vi "BRig_Host__Loop_Producer__tcp_System__Data_v2.vi"(0 "input_strCmd":string) -> ()   [LabVIEW 2014]
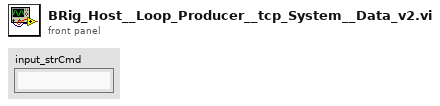
[diagram p1: front panel]
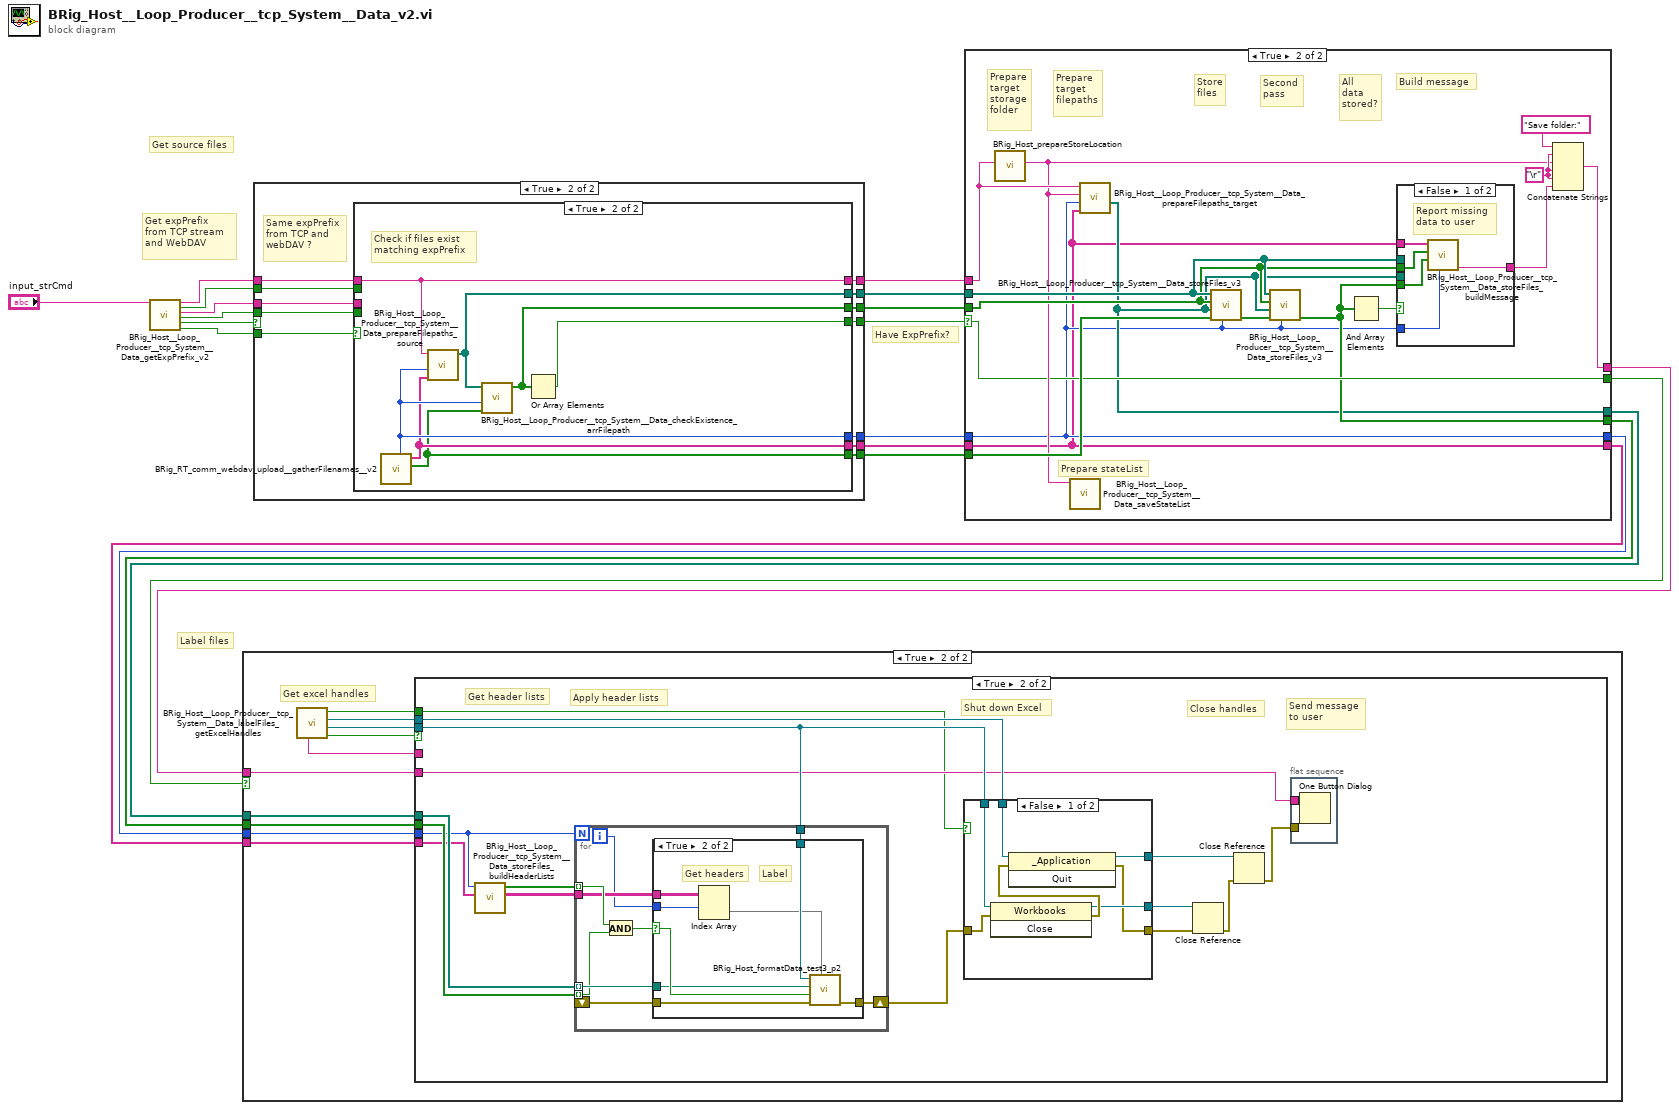
[diagram p0: block diagram]
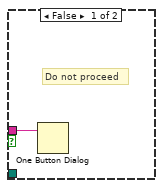
[diagram p2: hidden frame]
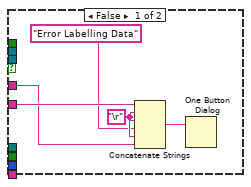
[diagram p3: hidden frame]
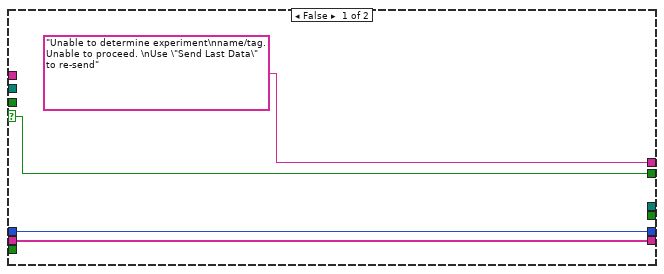
[diagram p6: hidden frame]
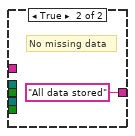
[diagram p7: hidden frame]
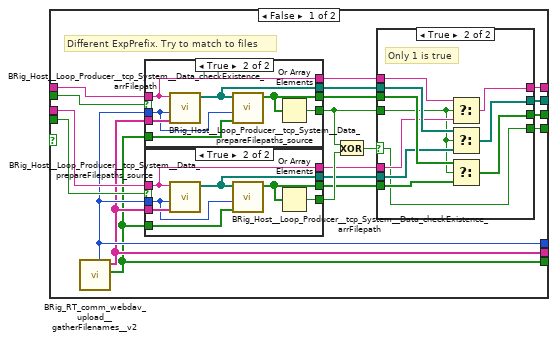
[diagram p9: hidden frame]
diagram:
  # "Label files"
  # "Have ExpPrefix?"
  # "Get expPrefix\nfrom TCP stream\nand WebDAV"
  # "Get source files"
  n1 = call "BRig_Host__Loop_Producer__tcp_System__Data_getExpPrefix_v2.vi"("input_strCmd"="input_strCmd") -> (14:"output_expPrefix_tcp"=w14:string, 15:"output_expPrefix_tcp"=w15:bool, 16:"output_expPrefix_webdav"=w16:string, 17:"output_expPrefix_webdav"=w17:bool, "output_expPrefix_any"=w19:bool, "output_expPrefix_same"=w18:bool)  [unwired: 13 in]
  n2 = case shown="True" w19 {
    tunnel: w18 -> [_ w32]
    tunnel: w17 -> [_ w28]
    tunnel: w16 -> [_ w30]
    tunnel: w15 -> [_ w29]
    tunnel: w14 -> [_ w31]
    tunnel: [_ w27] -> w12
    tunnel: [_ w26] -> w11
    tunnel: [_ w25] -> w10
    tunnel: [_ w24] -> w13
    tunnel: [_ w23] -> w9
    tunnel: [_ w22] -> w8
    tunnel: [_ w21] -> w7
    frame False {
    }
    frame True {
      # "Same expPrefix\nfrom TCP and\nwebDAV ?"
      n3 = case shown="True" w32 {
        tunnel: w31 -> [w51 w84]
        tunnel: w30 -> [w50 _]
        tunnel: w29 -> [w52 _]
        tunnel: w28 -> [w49 _]
        tunnel: [w39 w84] -> w27
        tunnel: [w38 w83] -> w26
        tunnel: [w37 w82] -> w25
        tunnel: [w36 w81] -> w24
        tunnel: [w35 w80] -> w23
        tunnel: [w34 w79] -> w22
        tunnel: [w33 w78] -> w21
        frame False {
          # "Different ExpPrefix. Try to match to files"
          n4 = call "BRig_RT_comm_webdav_upload__gatherFilenames__v2.vi"() -> ("output_arrBlank"=w33:bool[], "output_arrFilenames"=w34:string[], "output_n"=w35:i32)  [unwired: 9 in]
          n5 = case shown="True" w52 {
            tunnel: w51 -> [_ w74]
            tunnel: w35 -> [_ w76]
            tunnel: w34 -> [_ w77]
            tunnel: w33 -> [_ w75]
            tunnel: [_ w74] -> w46
            tunnel: [_ w73] -> w45
            tunnel: [_ w72] -> w44
            tunnel: [_ w71] -> w40
            frame False {
            }
            frame True {
              n6 = call "BRig_Host__Loop_Producer__tcp_System__Data_prepareFilepaths_source.vi"("input_arrFilenames"=w77, "input_nFilenames"=w76, "input_expPrefix"=w74) -> ("output_arrPath"=w73:path[])  [unwired: 8 in]
              n7 = call "BRig_Host__Loop_Producer__tcp_System__Data_checkExistence_arrFilepath.vi"("input_I_arrPath"=w75, "input_n"=w76, "input_arrPath"=w73) -> ("output_exist"=w72:bool[])  [unwired: 8 in]
              n8 = Or Array Elements(Boolean array=w72) -> (logical OR=w71:bool)
            }
          }
          n9 = case shown="True" w49 {
            tunnel: w50 -> [_ w67]
            tunnel: w35 -> [_ w69]
            tunnel: w34 -> [_ w70]
            tunnel: w33 -> [_ w68]
            tunnel: [_ w67] -> w43
            tunnel: [_ w66] -> w42
            tunnel: [_ w65] -> w41
            tunnel: [_ w64] -> w48
            frame False {
            }
            frame True {
              n10 = call "BRig_Host__Loop_Producer__tcp_System__Data_prepareFilepaths_source.vi"("input_arrFilenames"=w70, "input_nFilenames"=w69, "input_expPrefix"=w67) -> ("output_arrPath"=w66:path[])  [unwired: 8 in]
              n11 = call "BRig_Host__Loop_Producer__tcp_System__Data_checkExistence_arrFilepath.vi"("input_I_arrPath"=w68, "input_n"=w69, "input_arrPath"=w66) -> ("output_exist"=w65:bool[])  [unwired: 8 in]
              n12 = Or Array Elements(Boolean array=w65) -> (logical OR=w64:bool)
            }
          }
          n13 = Exclusive Or(1:w48, 2:w40) -> (0:w47:bool)
          n14 = case shown="True" w47 {
            selector: w47 -> [_ w53]
            tunnel: w46 -> [_ w63]
            tunnel: w45 -> [_ w62]
            tunnel: w44 -> [_ w61]
            tunnel: w43 -> [_ w60]
            tunnel: w42 -> [_ w59]
            tunnel: w41 -> [_ w58]
            tunnel: w40 -> [_ w57]
            tunnel: [_ w56] -> w39
            tunnel: [_ w55] -> w38
            tunnel: [_ w54] -> w37
            tunnel: [_ w53] -> w36
            frame False {
              # "Both false or both true\n\nIf false, can't proceed\nIf true, no way to choose"
            }
            frame True {
              # "Only 1 is true"
              n15 = Select(t=w63, s=w57, f=w60) -> (s? t:f=w56:string)
              n16 = Select(t=w62, s=w57, f=w59) -> (s? t:f=w55:path[])
              n17 = Select(t=w61, s=w57, f=w58) -> (s? t:f=w54:bool[])
            }
          }
        }
        frame True {
          # "Check if files exist\nmatching expPrefix"
          n18 = call "BRig_RT_comm_webdav_upload__gatherFilenames__v2.vi"() -> ("output_arrBlank"=w78:bool[], "output_arrFilenames"=w79:string[], "output_n"=w80:i32)  [unwired: 9 in]
          n19 = call "BRig_Host__Loop_Producer__tcp_System__Data_prepareFilepaths_source.vi"("input_arrFilenames"=w79, "input_nFilenames"=w80, "input_expPrefix"=w84) -> ("output_arrPath"=w83:path[])  [unwired: 8 in]
          n20 = call "BRig_Host__Loop_Producer__tcp_System__Data_checkExistence_arrFilepath.vi"("input_I_arrPath"=w78, "input_n"=w80, "input_arrPath"=w83) -> ("output_exist"=w82:bool[])  [unwired: 8 in]
          n21 = Or Array Elements(Boolean array=w82) -> (logical OR=w81:bool)
        }
      }
    }
  }
  n22 = case shown="True" w13 {
    selector: w13 -> [w87 w93]
    tunnel: w12 -> [_ w104]
    tunnel: w11 -> [_ w100]
    tunnel: w10 -> [_ w99]
    tunnel: w9 -> [w85 w90]
    tunnel: w8 -> [w86 w89]
    tunnel: w7 -> [_ w103]
    tunnel: ["Unable to determine experiment\nname/tag. Unable to proceed. \nUse \"Send Last Data\" to re-send" ("message") w94] -> w3
    tunnel: [w87 w93] -> w4
    tunnel: [_ w92] -> w6
    tunnel: [_ w91] -> w5
    tunnel: [w85 w90] -> w2
    tunnel: [w86 w89] -> w1
    frame False {
    }
    frame True {
      w98 = "\r"
      # "Build message"
      # "All\ndata\nstored?"
      # "Second\npass"
      # "Store\nfiles"
      # "Prepare stateList"
      # "Prepare\ntarget\nstorage\nfolder"
      # "Prepare\ntarget\nfilepaths"
      n23 = call "BRig_Host_prepareStoreLocation.vi"("input_expPrefix"=w104) -> ("output_folderPath"=w97:string)  [unwired: 9 in, 1 out]
      n24 = call "BRig_Host__Loop_Producer__tcp_System__Data_saveStateList.vi"("input_filepath_storage"=w97) -> ()  [unwired: 11 in]
      n25 = call "BRig_Host__Loop_Producer__tcp_System__Data_prepareFilepaths_target.vi"("input_arrFilenames"=w89, "input_nFilenames"=w90, "input_storagePath"=w97, "input_expPrefix"=w104) -> ("output_arrPath_target"=w91:path[])  [unwired: 7 in]
      n26 = call "BRig_Host__Loop_Producer__tcp_System__Data_storeFiles_v3.vi"("input_n"=w90, "input_stored"=w103, "input_arrPath_target"=w91, "input_exist_source"=w99, "input_arrPath_source"=w100) -> ("output_stored"=w102:bool[])  [unwired: 6 in]
      n27 = call "BRig_Host__Loop_Producer__tcp_System__Data_storeFiles_v3.vi"("input_n"=w90, "input_stored"=w102, "input_arrPath_target"=w91, "input_exist_source"=w99, "input_arrPath_source"=w100) -> ("output_stored"=w92:bool[])  [unwired: 6 in]
      n28 = And Array Elements(Boolean array=w92) -> (logical AND=w101:bool)
      n29 = case shown="False" w101 {
        tunnel: w100 -> [_ _]
        tunnel: w99 -> [w108 _]
        tunnel: w91 -> [_ _]
        tunnel: w92 -> [w107 _]
        tunnel: w89 -> [w109 _]
        tunnel: w90 -> [w106 _]
        tunnel: [w105 "All data stored" ("output_msg")] -> w95
        frame False {
          # "Report missing\ndata to user"
          n30 = call "BRig_Host__Loop_Producer__tcp_System__Data_storeFiles_buildMessage.vi"("input_n"=w106, "input_stored"=w107, "input_exist_source"=w108, "input_arrFilenames"=w109) -> ("output_msg"=w105:string)  [unwired: 7 in]
        }
        frame True {
          # "No missing data"
        }
      }
      n31 = Concatenate Strings("Save folder:" ("string"), w98, w97, w98, w98, w95) -> (w94:string)
    }
  }
  n32 = case shown="True" w4 {
    tunnel: w6 -> [_ w114]
    tunnel: w5 -> [_ w113]
    tunnel: w3 -> [w111 w112]
    tunnel: w2 -> [_ w116]
    tunnel: w1 -> [_ w115]
    frame False {
      # "Do not proceed"
      n33 = One Button Dialog(message=w111) -> ()  [unwired: 1 in, 1 out]
    }
    frame True {
      # "Get excel handles"
      n34 = call "BRig_Host__Loop_Producer__tcp_System__Data_labelFiles_getExcelHandles.vi"() -> ("output_hExcel"=w121:bool, "output_hExcel_Workbooks"=w120:refnum<k7>, "output_hExcel_Application"=w119:refnum<k7>, "output_excel_runningPreviously"=w118:bool, "output_haveErrorMsg"=w117:string)  [unwired: 7 in]
      n35 = case shown="True" w121 {
        tunnel: w120 -> [_ w139]
        tunnel: w119 -> [_ w138]
        tunnel: w118 -> [_ w127]
        tunnel: w117 -> [w123 _]
        tunnel: w116 -> [_ w130]
        tunnel: w115 -> [_ w131]
        tunnel: w114 -> [_ w142]
        tunnel: w113 -> [_ w141]
        tunnel: w112 -> [w126 w132]
        frame False {
          w124 = "\r"
          n36 = Concatenate Strings(w126, w124, w124, "Error Labelling Data" ("string"), w124, w123) -> (w125:string)
          n37 = One Button Dialog(message=w125) -> ()  [unwired: 1 in, 1 out]
        }
        frame True {
          # "Send message\nto user"
          # "Close handles"
          # "Shut down Excel"
          # "Apply header lists"
          # "Get header lists"
          n38 = call "BRig_Host__Loop_Producer__tcp_System__Data_storeFiles_buildHeaderLists.vi"("input_arrFilenames"=w131, "input_nFilenames"=w130) -> (2:"output_HeaderLists"=w128:string[][], 3:"output_HeaderLists"=w129:bool[])  [unwired: 8 in]
          n39 = for {
            N: w130 -> [_]
            tunnel: w139 -> [w162]
            shift-right: [w161] -> w140
            shift-left: _ -> [w160]
            tunnel: w142 -> [w157] mode=indexing
            tunnel: w141 -> [w159] mode=indexing
            tunnel: w129 -> [w158] mode=indexing
            tunnel: w128 -> [w155]
            i -> [w154]
            n40 = And(x=w158, y=w157) -> (x .and. y?=w156:bool)
            n41 = case shown="True" w156 {
              selector: w156 -> [_ w168]
              tunnel: w162 -> [_ w171]
              tunnel: [w163 w170] -> w161
              tunnel: w160 -> [w163 w169]
              tunnel: w159 -> [_ w167]
              tunnel: w155 -> [_ w166]
              tunnel: w154 -> [_ w165]
              frame False {
              }
              frame True {
                # "Label"
                # "Get headers"
                n42 = Index Array(array=w166, index (row)=w165) -> (element=w164:string[])  [unwired: 1 in]
                n43 = call "BRig_Host_formatData_test3_p2.vi"("input_headers"=w164, "input_error"=w169, "input_Iexist"=w168, "input_filePath"=w167, "input_hdl_Workbooks"=w171) -> ("output_error"=w170:errorcluster)  [unwired: 4 in, 2 out]
              }
            }
          }
          n44 = case shown="False" w127 {
            tunnel: w140 -> [w149 w150]
            tunnel: w139 -> [w148 w151]
            tunnel: w138 -> [w146 w152]
            tunnel: [w145 w151] -> w137
            tunnel: [w144 w150] -> w136
            tunnel: [w143 w152] -> w135
            frame False {
              n45 = invoke class="Workbooks" method="Close"(reference=w148, error in=w149) -> (reference out=w145:refnum<k7>, error out=w147:errorcluster)  [unwired: 1 in, 1 out]
              n46 = invoke class="_Application" method="Quit"(reference=w146, error in=w147) -> (reference out=w143:refnum<k7>, error out=w144:errorcluster)  [unwired: 1 in, 1 out]
            }
            frame True {
            }
          }
          n47 = Close Reference(reference=w137, error in (no error)=w136) -> (error out=w134:errorcluster)
          n48 = Close Reference(reference=w135, error in (no error)=w134) -> (error out=w133:errorcluster)
          n49 = flat-sequence {
            tunnel: w133 -> [_]
            tunnel: w132 -> [w153]
            frame #0 {
              n50 = One Button Dialog(message=w153) -> ()  [unwired: 1 in, 1 out]
            }
          }
        }
      }
    }
  }
